vi "ClosePort.vi"(1 "Serial port":refnum<visa-resource-name>) -> ()   [LabVIEW 2021]
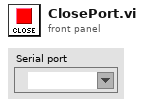
[diagram p1: front panel]
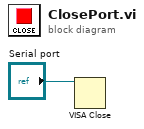
[diagram p0: block diagram]
diagram:
  n1 = VISA Close(VISA resource name="Serial port") -> ()  [unwired: 1 in, 1 out]
